vi "switchToCamRam.vi"(0 "Camera in":refnum<class "Camera.lvclass">, 5 "segment":u16=65535, 11 "error in (no error)":errorcluster) -> (4 "Camera out":refnum<class "Camera.lvclass">, 15 "error out":errorcluster)   [LabVIEW 2019, in "Camera.lvclass"]
doc: "Switch the active RAM segment in cameras with internal memory (CAMRAM)."
uses:
  Camera.lvclass
  Camera.lvclass/Camera.ctl
  pco.sdk/RecordingControl/RecordingControl.lvlib
  pco.sdk/StorageControl/StorageControl.lvlib
  pco.recorder/Recorder.lvlib
  pco.convert/Convert.lvlib
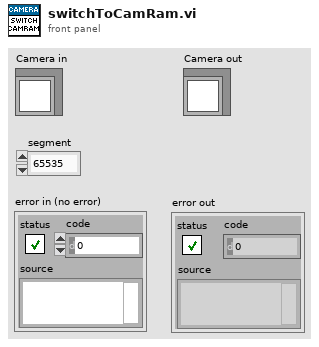
[diagram p1: front panel]
types:
  T1 = cluster{"iConversionFactor":i32, "iDataBits":i32, "iSensorInfoBits":i32, "iDarkOffset":i32, "strColorCoeff":dbl[], "iCamNum":i32, "hCamera":u64}
  T2 = map{enum16{"Undefined", "Mono8", "Mono16", "BGRA8", "RGBA8", "BGRA16", "RGBA16", "CompressedMono8"}, u64}
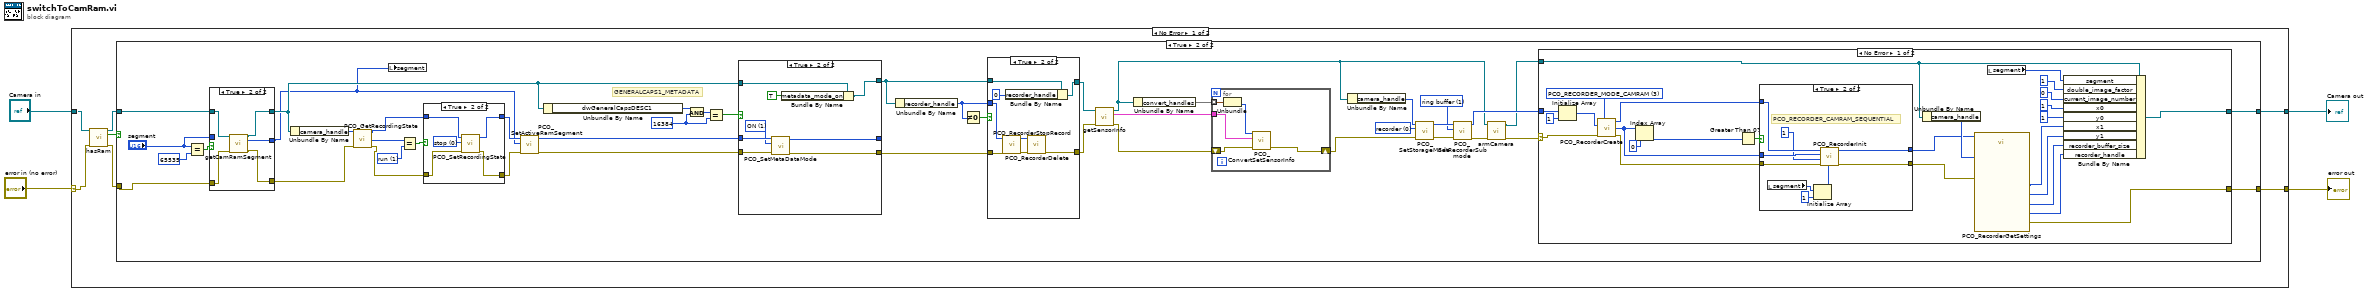
[diagram p0: block diagram]
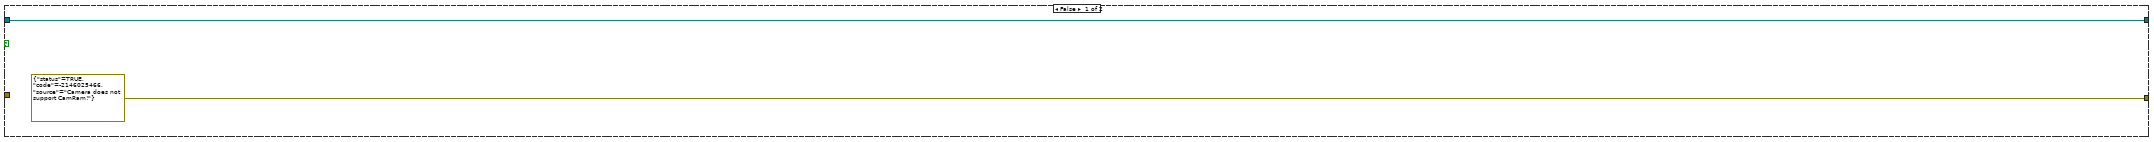
[diagram p2: hidden frame]
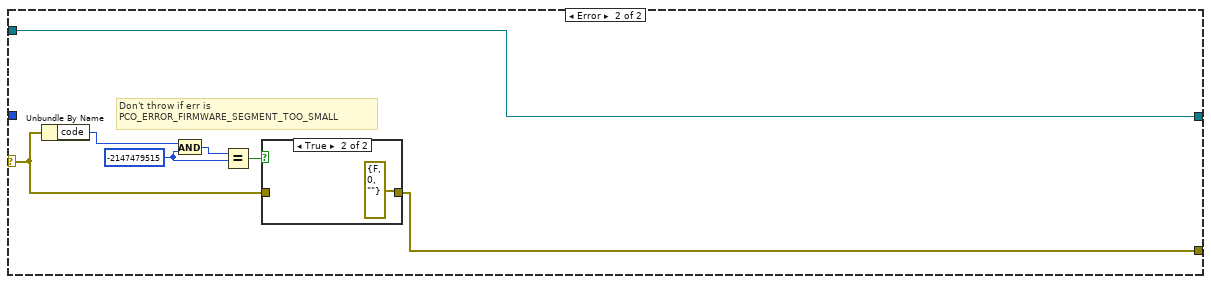
[diagram p4: hidden frame]
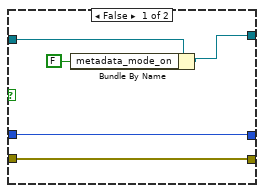
[diagram p7: hidden frame]
diagram:
  n1 = case shown="No Error" "error in (no error)" {
    selector: "error in (no error)" -> [w10 w148]
    tunnel: [w6 w148] -> w2
    tunnel: [w5 w147] -> w3
    tunnel: "Camera in" -> [w8 w147]
    frame No Error {
      n2 = call-dynamic "hasRam.vi"("Camera in"=w8, "error in (no error)"=w10) -> ("Camera out"=w7:refnum<class "Camera.lvclass">, "hasRam"=w11:bool, "error out"=w9:errorcluster)  [unwired: 11 in]
      n3 = case shown="True" w11 {
        tunnel: w7 -> [w12 w54]
        tunnel: w9 -> [_ w53]
        tunnel: [errorcluster {"status"=TRUE, "code"=-2146025466, "source"="Camera does not support CamRam!"} ("error constant") w19] -> w6
        tunnel: [w12 w20] -> w5
        frame False {
        }
        frame True {
          w22 = u16 1 items=["sequence", "ring buffer"] ("wRecSubmode")
          w26 = u16 0 items=["recorder", "FIFO buffer"] ("wStorageMode")
          w42 = u32 16384 ("y")
          w49 = u16 1 items=["stop", "run"] ("wRecState")
          # "GENERALCAPS1_METADATA"
          n4 = Equal?(x="segment", y=u16 65535) -> (x = y?=w56:bool)
          n5 = case shown="True" w56 {
            tunnel: "segment" -> [w139 _]
            tunnel: w54 -> [w141 w146]
            tunnel: w53 -> [w140 w145]
            tunnel: [w139 w144] -> w18
            tunnel: [w141 w143] -> w40
            tunnel: [w140 w142] -> w51
            frame False {
            }
            frame True {
              n6 = call-dynamic "getCamRamSegment.vi"("Camera in"=w146, "error in (no error)"=w145) -> ("Camera out"=w143:refnum<class "Camera.lvclass">, "segment"=w144:u16, "error out"=w142:errorcluster)  [unwired: 11 in]
            }
          }
          n7 = Unbundle By Name(w40) -> ("camera_handle"=w52:u64)
          n8 = call "PCO_GetRecordingState.vi"("error in (no error)"=w51, "ph"=w52) -> ("error out"=w47:errorcluster, "wRecState"=w50:u16, "ph out"=w46:u64)  [unwired: 6 in, 1 out]
          n9 = local write "segment"(w18) -> ()
          n10 = Equal?(x=w50, y=w49) -> (x = y?=w48:bool)
          n11 = case shown="True" w48 {
            tunnel: w47 -> [w132 w136]
            tunnel: w46 -> [w133 w137]
            tunnel: [w132 w135] -> w44
            tunnel: [w133 w134] -> w45
            frame False {
            }
            frame True {
              w138 = u16 0 items=["stop", "run"] ("wRecState")
              n12 = call "PCO_SetRecordingState.vi"("error in (no error)"=w136, "wRecState"=w138, "ph"=w137) -> ("error out"=w135:errorcluster, "ph out"=w134:u64)  [unwired: 6 in, 1 out]
            }
          }
          n13 = call "PCO_SetActiveRamSegment.vi"("error in (no error)"=w44, "wActSeg"=w18, "ph"=w45) -> ("error out"=w37:errorcluster, "ph out"=w38:u64)  [unwired: 6 in, 1 out]
          n14 = Unbundle By Name(w40) -> ("dwGeneralCapsDESC1"=w41:u32)
          n15 = And(x=w41, y=w42) -> (x .and. y?=w43:u32)
          n16 = Equal?(x=w43, y=w42) -> (x = y?=w39:bool)
          n17 = case shown="True" w39 {
            tunnel: w40 -> [w123 w127]
            tunnel: [w121 w126] -> w33
            tunnel: w38 -> [w120 w131]
            tunnel: w37 -> [w119 w130]
            tunnel: [w119 w125] -> w34
            tunnel: [w120 w124] -> _
            frame False {
              n18 = Bundle By Name(cluster=w123, "metadata_mode_on"=FALSE) -> (w121:refnum<class "Camera.lvclass">)
            }
            frame True {
              w129 = u16 1 items=["OFF", "ON"] ("wMetaDataMode")
              n19 = call "PCO_SetMetaDataMode.vi"("error in (no error)"=w130, "wMetaDataMode"=w129, "ph"=w131) -> ("error out"=w125:errorcluster, "ph out"=w124:u64)  [unwired: 4 in, 3 out]
              n20 = Bundle By Name(cluster=w127, "metadata_mode_on"=TRUE) -> (w126:refnum<class "Camera.lvclass">)
            }
          }
          n21 = Unbundle By Name(w33) -> ("recorder_handle"=w35:u64)
          n22 = Not Equal To 0?(x=w35) -> (x != 0?=w36:bool)
          n23 = case shown="True" w36 {
            tunnel: w35 -> [_ w117]
            tunnel: w34 -> [w109 w118]
            tunnel: w33 -> [w110 w114]
            tunnel: [w110 w112] -> w32
            tunnel: [w109 w111] -> w31
            frame False {
            }
            frame True {
              n24 = call "PCO_RecorderStopRecord.vi"("error in (no error)"=w118, "phRec"=w117) -> ("error out"=w116:errorcluster, "phRec out"=w115:u64)  [unwired: 7 in, 1 out]
              n25 = Bundle By Name(cluster=w114, "recorder_handle"=u64 0) -> (w112:refnum<class "Camera.lvclass">)
              n26 = call "PCO_RecorderDelete.vi"("error in (no error)"=w116, "phRec"=w115) -> ("error out"=w111:errorcluster)  [unwired: 8 in, 1 out]
            }
          }
          n27 = call-dynamic "getSensorInfo.vi"("error in (no error)"=w31, "Camera in"=w32) -> ("error out"=w28:errorcluster, "PCO_SensorInfo"=w29:T1, "Camera out"=w16:refnum<class "Camera.lvclass">)  [unwired: 7 in]
          n28 = Unbundle By Name(w16) -> ("convert_handles"=w30:T2)
          n29 = for {
            tunnel: w30 -> [w107] mode=indexing
            tunnel: w29 -> [w108]
            shift-right: [w104] -> w27
            shift-left: w28 -> [w105]
            n30 = Unbundle(w107) -> (w106:u64)  [unwired: 1 out]
            n31 = call "PCO_ConvertSetSensorInfo.vi"("error in (no error)"=w105, "strSensorInfo"=w108, "ph"=w106) -> ("error out"=w104:errorcluster)  [unwired: 6 in, 2 out]
          }
          n32 = Unbundle By Name(w16) -> ("camera_handle"=w25:u64)
          n33 = call "PCO_SetStorageMode.vi"("error in (no error)"=w27, "wStorageMode"=w26, "ph"=w25) -> ("error out"=w23:errorcluster, "ph out"=w24:u64)  [unwired: 6 in, 1 out]
          n34 = call "PCO_SetRecorderSubmode.vi"("error in (no error)"=w23, "wRecSubmode"=w22, "ph"=w24) -> ("error out"=w21:errorcluster, "ph out"=w17:u64)  [unwired: 6 in, 1 out]
          n35 = call-dynamic "armCamera.vi"("Camera in"=w16, "error in (no error)"=w21) -> ("Camera out"=w15:refnum<class "Camera.lvclass">, "error out"=w14:errorcluster)  [unwired: 12 in]
          n36 = case shown="No Error" w14 {
            selector: w14 -> [w58 w96]
            tunnel: w17 -> [w83 _]
            tunnel: [w62 w98] -> w19
            tunnel: [w61 w97] -> w20
            tunnel: w15 -> [w64 w97]
            frame No Error {
              w80 = u16 3 items=["PCO_RECORDER_MODE_FILE"=1, "PCO_RECORDER_MODE_MEMORY"=2, "PCO_RECORDER_MODE_CAMRAM"=3] ("wRecMode")
              n37 = Initialize Array(w83, 1 ("dimension size")) -> (w81:u64[])
              n38 = call "PCO_RecorderCreate.vi"("wRecMode"=w80, "phCamArr"=w81, "error in (no error)"=w58) -> ("phRec out"=w76:u64, "dwMaxImgCountArr"=w74:u32[], "error out"=w75:errorcluster)  [unwired: 9 in, 1 out]
              n39 = Index Array(array=w74, index=0) -> (element=w78:u32)
              n40 = Greater Than 0?(x=w78) -> (x > 0?=w77:bool)
              n41 = case shown="True" w77 {
                tunnel: w76 -> [w84 w93]
                tunnel: w75 -> [w85 w94]
                tunnel: w74 -> [_ w92]
                tunnel: [w85 w88] -> w73
                tunnel: [w84 w87] -> w60
                frame False {
                }
                frame True {
                  # "PCO_RECORDER_CAMRAM_SEQUENTIAL"
                  n42 = local read "segment"() -> (w90:u16)
                  n43 = Initialize Array(w90, 1 ("dimension size")) -> (w89:u16[])
                  n44 = call "PCO_RecorderInit.vi"("wRamSegmentArr"=w89, "error in (no error)"=w94, "wType"=u16 1, "dwImgCountArr"=w92, "phRec"=w93) -> ("error out"=w88:errorcluster, "phRec out"=w87:u64)  [unwired: 4 in, 1 out]
                }
              }
              n45 = Unbundle By Name(w64) -> ("camera_handle"=w72:u64)
              n46 = call "PCO_RecorderGetSettings.vi"("phRec"=w60, "phCam"=w72, "error in (no error)"=w73) -> ("wHeight"=w65:u16, "phRec out"=w63:u64, "dwMaxImgCount"=w69:u32, "wWidth"=w66:u16, "error out"=w62:errorcluster)  [unwired: 4 in, 4 out]
              n47 = local read "segment"() -> (w59:u16)
              n48 = Bundle By Name(cluster=w64, "segment"=w59, "double_image_factor"=u16 1, "current_image_number"=u32 0, "x0"=u64 1 ("hard_roi.x0"), "y0"=u64 1 ("hard_roi.x0"), "x1"=w66, "y1"=w65, "recorder_buffer_size"=w69, "recorder_handle"=w63) -> (w61:refnum<class "Camera.lvclass">)
            }
            frame Error {
              w100 = -2147479515 ("y")
              # "Don't throw if err is\nPCO_ERROR_FIRMWARE_SEGMENT_TOO_SMALL"
              n49 = Unbundle By Name(w96) -> ("code"=w95:i32)
              n50 = And(x=w95, y=w100) -> (x .and. y?=w101:i32)
              n51 = Equal?(x=w101, y=w100) -> (x = y?=w99:bool)
              n52 = case shown="True" w99 {
                tunnel: w96 -> [w102 _]
                tunnel: [w102 errorcluster {"status"=FALSE, "code"=0, "source"=""} ("error out")] -> w98
                frame False {
                }
                frame True {
                }
              }
            }
          }
        }
      }
    }
    frame Error {
    }
  }
  "error out" <- w2
  "Camera out" <- w3
